vi "Build Bulk Create.vi"(8 "error in (no error)":errorcluster, 9 "tableName":string, 10 "DynamicParameters in":refnum<class "DynamicParameters.lvclass">[](array[class]), 11 "SQLConnection in":refnum<class "DBC.lvclass">) -> (0 "error out":errorcluster, 2 "BulkInsertQuery":string, 3 "SQLConnection out":refnum<class "DBC.lvclass">)   [LabVIEW 2020, in "ORM_DBC_Mssql.lvlib" / "DBC.lvclass"]
uses:
  DBC.lvclass
  <vilib>/Viviota/shared/ORM.lvlibp/ORM/DynamicParameters/DynamicParameters.lvclass
  <vilib>/Viviota/shared/ORM.lvlibp/ORM/DynamicParameters/Read AutoKey.vi
  <vilib>/Viviota/shared/ORM.lvlibp/ORM/DbConnection/DbConnection.lvclass
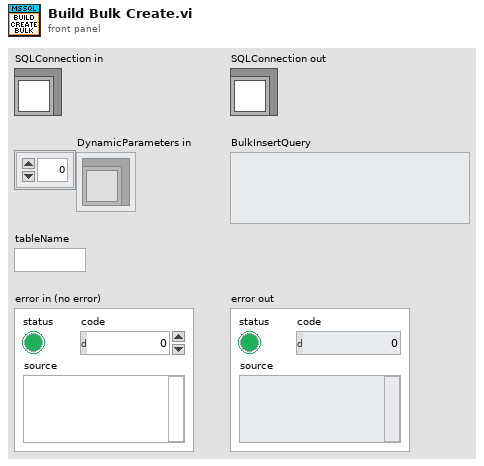
[diagram p1: front panel]
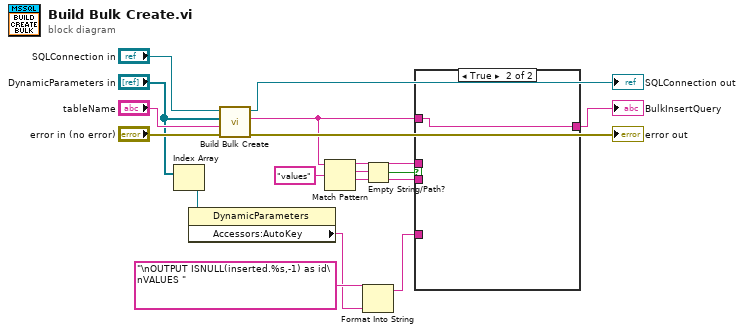
[diagram p0: block diagram]
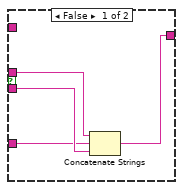
[diagram p2: hidden frame]
diagram:
  n1 = Index Array(array="DynamicParameters in") -> (element=w1:refnum<class "DynamicParameters.lvclass">)  [unwired: 1 in]
  n2 = property class="DynamicParameters"(reference=w1) -> ("Accessors:AutoKey"=w7:string)  [unwired: 1 in, 2 out]
  n3 = call-parent "Build Bulk Create.vi"("error in (no error)"="error in (no error)", "tableName"="tableName", "DynamicParameters in"="DynamicParameters in", "DbConnection in"="SQLConnection in") -> ("error out"=→"error out":errorcluster, "BulkInsertQuery"=w4:string, "DbConnection out"=→"SQLConnection out":refnum<class "DBC.lvclass">)  [unwired: 5 in]
  n4 = Match Pattern(string=w4, regular expression="values") -> (before substring=w10:string, match substring=w12:string, after substring=w9:string)  [unwired: 1 in, 1 out]
  n5 = Empty String/Path?(string/path=w12) -> (empty?=w11:bool)
  n6 = Format Into String(format string="\nOUTPUT ISNULL(inserted.%s,-1) as id\nVALUES " ("string"), w7) -> (resulting string=w6:string)  [unwired: 2 in, 1 out]
  n7 = case shown="True" w11 {
    tunnel: w4 -> [_ w22]
    tunnel: [w18 w22] -> w3
    tunnel: w10 -> [w19 _]
    tunnel: w9 -> [w21 _]
    tunnel: w6 -> [w20 _]
    frame False {
      n8 = Concatenate Strings(w19, w20, w21) -> (w18:string)
    }
    frame True {
    }
  }
  "BulkInsertQuery" <- w3
